vi "FPGAmain_v2.vi"() -> ()   [LabVIEW 2013]
uses:
  FPGA/DataMode.ctl
  FPGA/AcquireState.ctl
  FPGA/Input_5782/5782_states.ctl
  <vilib>/Platform/TimedLoop/XDataNode/timing_clust.ctl
  <vilib>/Platform/TimedLoop/XDataNode/nitl_modes.ctl
  <vilib>/Platform/TimedLoop/XDataNode/wakeup.ctl
  <vilib>/rvi/Emulation/niFpgaSctlEmulationGetInTimedLoop.vi
  <vilib>/rvi/Emulation/niFpgaEmulationReportErrorSimple.vi
  <vilib>/rvi/Emulation/niFpgaGetClockAttributes.vi
  <vilib>/rvi/eio/common/nirviEmuTemplateMethod_errors.vi
  <vilib>/rvi/Emulation/niFpgaCriticalErrorInLSC.vi
  <vilib>/rvi/FIFO/Fifo_Resource/nirvififoEmulationWriteFpgaImpl.vi
  <vilib>/rvi/DataTransferAndStorage/Container/Common/niFpgaContainerGetUniqueNameForEmu.vi
  <vilib>/rvi/FIFO/Fifo_Resource/nirvififoEmulationReadFpgaImpl.vi
  <vilib>/rvi/DataTransferAndStorage/Register/Emulation/niFpgaRegisterEmulationFpgaImpl.vi
  <instcachedir>/0/niFpgaRegisterEmulationFpgaImpl_DCF4BC0110594B98B44A971D60CEEC4D.lvgen/niFpgaRegisterEmulationFpgaImpl_DCF4BC0110594B98B44A971D60CEEC4D_016.vi
  <instcachedir>/0/niFpgaRegisterEmulationFpgaImpl_DCF4BC0110594B98B44A971D60CEEC4D.lvgen/niFpgaRegisterEmulationFpgaImpl_DCF4BC0110594B98B44A971D60CEEC4D_003.vi
  <instcachedir>/0/niFpgaRegisterEmulationFpgaImpl_DCF4BC0110594B98B44A971D60CEEC4D.lvgen/niFpgaRegisterEmulationFpgaImpl_DCF4BC0110594B98B44A971D60CEEC4D_014.vi
  <instcachedir>/0/niFpgaRegisterEmulationFpgaImpl_DCF4BC0110594B98B44A971D60CEEC4D.lvgen/niFpgaRegisterEmulationFpgaImpl_DCF4BC0110594B98B44A971D60CEEC4D_015.vi
  <vilib>/rvi/interface/RandomDataEmulation/nirviRandomDataMultiElementFPGAFIFO.vi
  <instcachedir>/0/nirviRandomDataMultiElementFPGAFIFO_F2B80EDE0D7944A08478D8D26097D4DB.lvgen/nirviRandomDataMultiElementFPGAFIFO_F2B80EDE0D7944A08478D8D26097D4DB_005.vi
  <vilib>/rvi/interface/RandomDataEmulation/niFpgaRandomDataHandleErrors.vi
  <vilib>/rvi/interface/RandomDataEmulation/nirviRandomDataFPGAFIFO.vi
  <instcachedir>/0/niFpgaRegisterEmulationFpgaImpl_DCF4BC0110594B98B44A971D60CEEC4D.lvgen/niFpgaRegisterEmulationFpgaImpl_DCF4BC0110594B98B44A971D60CEEC4D_009.vi
  <instcachedir>/0/niFpgaRegisterEmulationFpgaImpl_DCF4BC0110594B98B44A971D60CEEC4D.lvgen/niFpgaRegisterEmulationFpgaImpl_DCF4BC0110594B98B44A971D60CEEC4D_013.vi
  <vilib>/Platform/TimedLoop/XDataNode/XDataNode.xnode
  <vilib>/eio/EIONode/EIONode.xnode
  <vilib>/rvi/DataTransferAndStorage/Container/XNode/niFpgaContainer.xnode
  <vilib>/rvi/FIFO/Fifo_Resource/nirvififoEmulationWrite.vi
  <vilib>/rvi/FIFO/Fifo_Resource/nirvififoEmulationRead.vi
  <vilib>/rvi/DataTransferAndStorage/Register/Emulation/niFpgaRegisterEmulation.vi
  <vilib>/rvi/interface/RandomDataEmulation/nirviRandomDataFpgaMultiElementTemplate.vi
  <vilib>/rvi/interface/RandomDataEmulation/nirviRandomDataFpgaReadWriteTemplate.vi
  <vilib>/rvi/FIFO/Fifo_Resource/nirvififoEmulationP2P.vi
  <vilib>/Platform/TimedLoop/XDataNode/XDNodeRunTimeDep.lvlib
  <instrlib>/FlexRIO/Libraries/Helper VIs/NI FlexRIO Helper VIs.lvlib
panel:
  in  "delay phase":fxp<+,64,64>
  in  "AM phase":fxp<+,64,64>
  in  "Phase 5782":fxp<+,64,64>[](array[numeric])=[0.0, 0.0]
  in  "User Command Commit":bool
  in  "User Command":u8
  out "User Command Idle":bool
  out "User Command Status":u8
  in  "User Data 0":u8
  in  "User Data 1":u8
  out "PLL Locked":bool
  out "User Error":bool
  out "Configured?":bool
  in  "FIR coeffs":fxp<+/-,18,18>[](array[numeric])
  in  "Phase output":fxp<+,64,64>[](array[numeric])=[0.0, 0.0, 0.0, 0.0]
  in  "5782 record length":u16=4000 caption="Samples Per Trigger" min=1 step=1
  in  "Trigger Acquisition":bool
  in  "Continuous":bool
  out "IO Module\\Trigger Input":bool
  in  "Mode":T1
  in  "Simulated phase 5782":fxp<+,64,64>[](array[numeric])=[0.0, 0.0]
  in  "Acquisition running":bool
  in  "Samples Per Trigger":i32 min=1 step=1
  in  "Trigger simulated data":bool
  in  "simulated phase 5160":fxp<+,64,64>
  in  "phase 5160":fxp<+,64,64>
  # "Dynamic filter"
  # "Dynamic downsample"
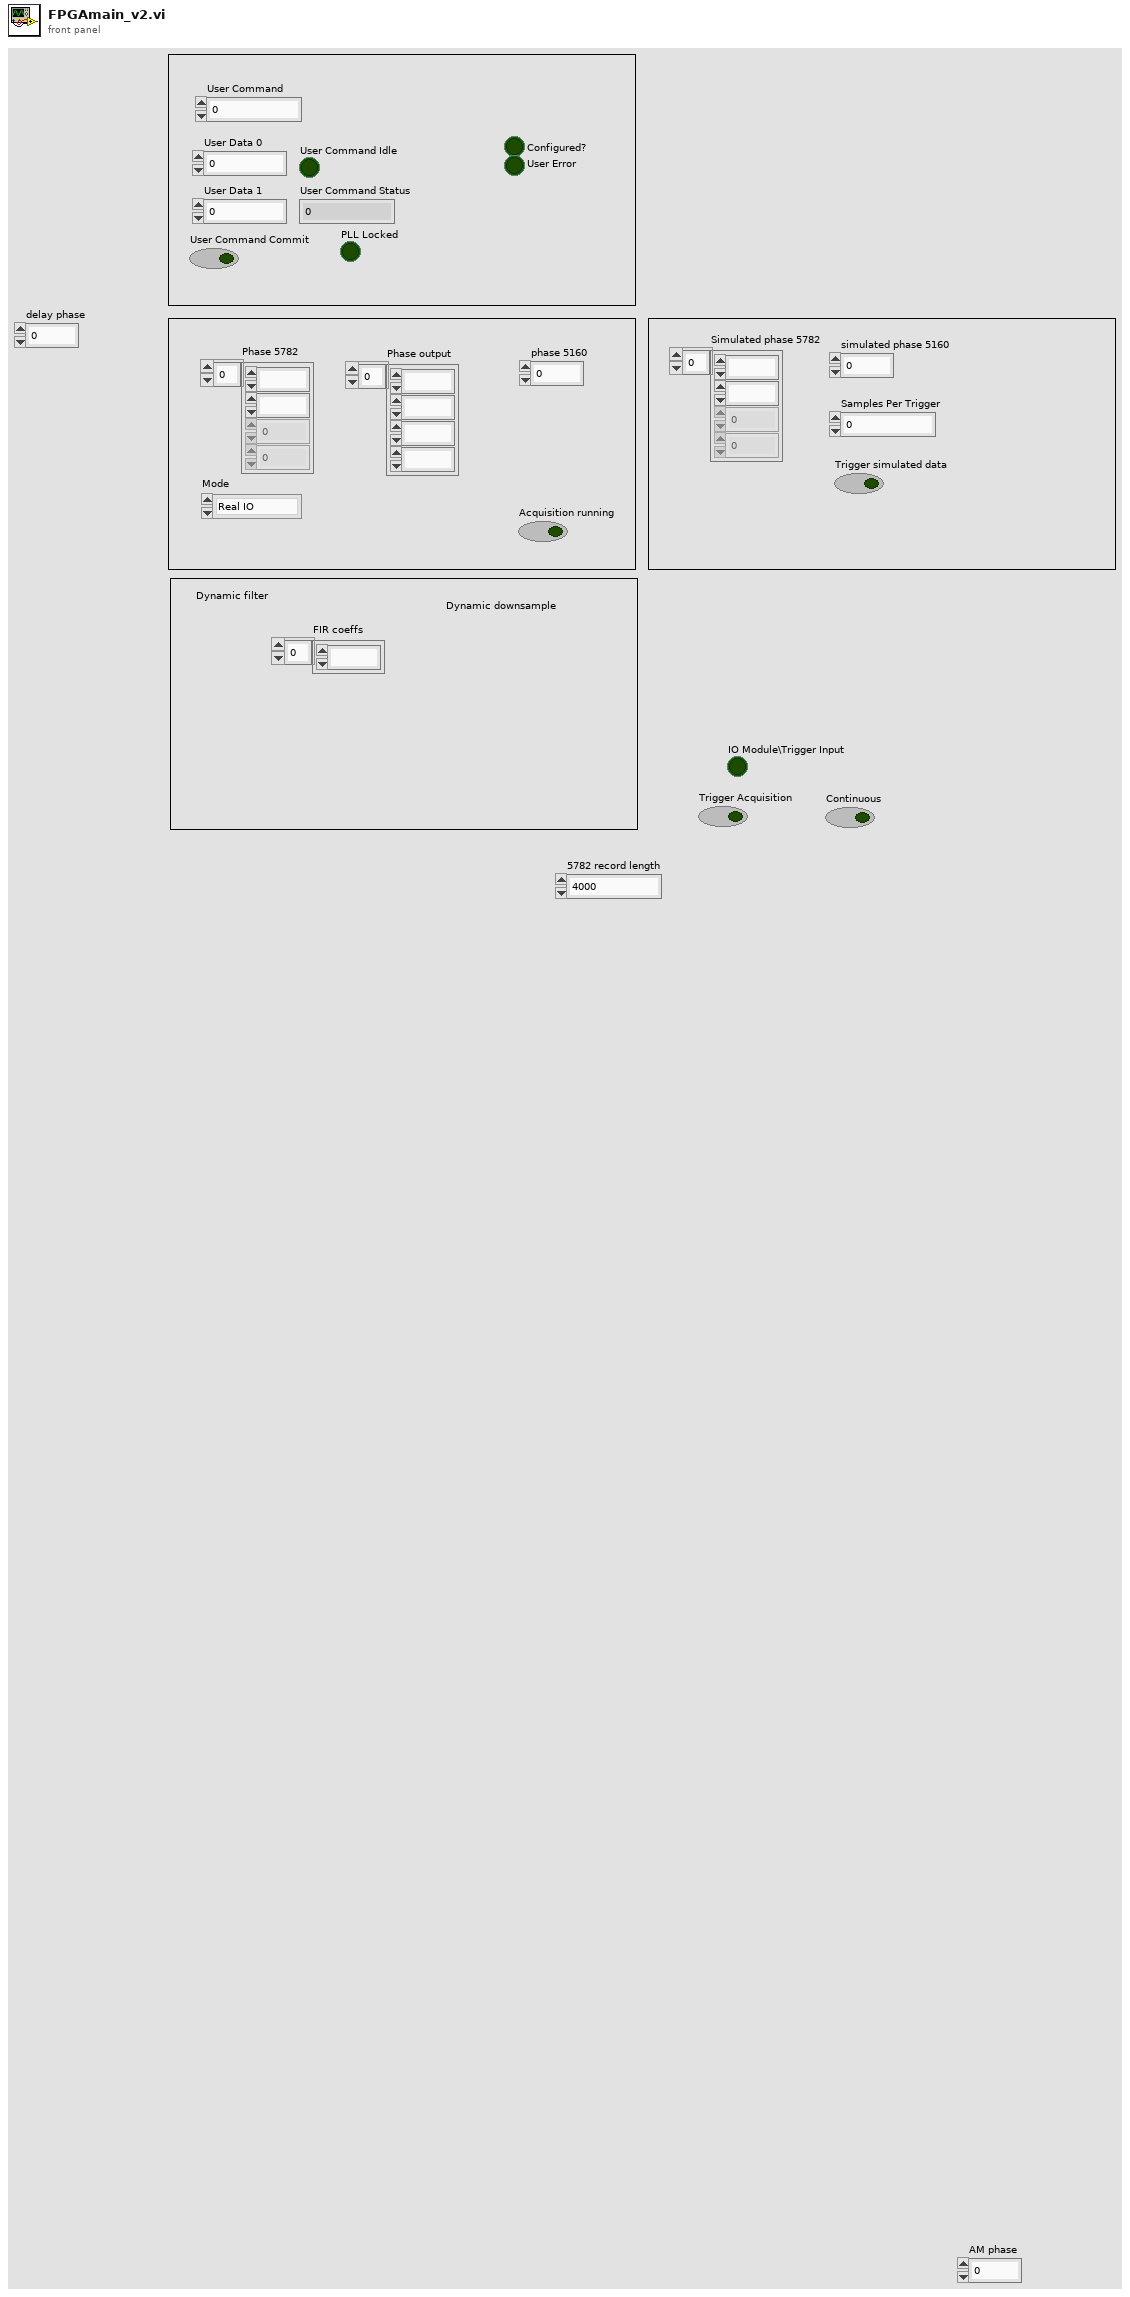
[diagram p1: front panel]
types:
  T1 = typedef "DataMode.ctl" = enum16{"Real IO", "Simulated"}
  T2 = typedef "5782_states.ctl" = enum8{"Wait for trigger", "Acquisition", "Send record length", "Quiet period"}
  T3 = typedef "AcquireState.ctl" = enum8{"Idle", "Acquire"}
  T4 = typedef "XDNodeRunTimeDep.lvlib/timing_clust.ctl" = cluster{"Expected End [f-1]":u64, "Actual End [f-1]":u64, "Finished Late? [f-1]":bool, "Expected End [i-1]":u64, "Actual End [i-1]":u64, "Finished Late? [i-1]":bool, "Expected Start [i]":u64, "Actual Start [i]":u64, "Expected Start [f]":u64, "Actual Start [f]":u64, "Source Name":string, "Structure Name":string, "Period":i64, "Deadline":i64, "Offset":i64, "Start":i64, "Priority":i32, "Timeout":i32, "Mode":T5, "Wakeup Reason":T6, "Error":errorcluster, "Source Type":string, "Secondary Source Type":string, "Global End Time":u64, "Global Start Time":u64, "Frame Duration":u64, "Iteration Duration":u64, "Assigned CPU":i32, "I/O Scan Engine Mode":u32}
  T5 = typedef "XDNodeRunTimeDep.lvlib/nitl_modes.ctl" = enum32{"No Change", "Process missed periods, maintain original phase", "Discard missed periods, maintain original phase", "Process missed periods, ignore original phase", "Discard missed periods, ignore original phase"}
  T6 = typedef "XDNodeRunTimeDep.lvlib/wakeup.ctl" = enum32{"Normal", "Aborted", "Asynchronous wakeup", "Timing source error", "Timed loop error", "Timeout"}
  T7 = typedef "I16 array size 2.ctl" = i16[]
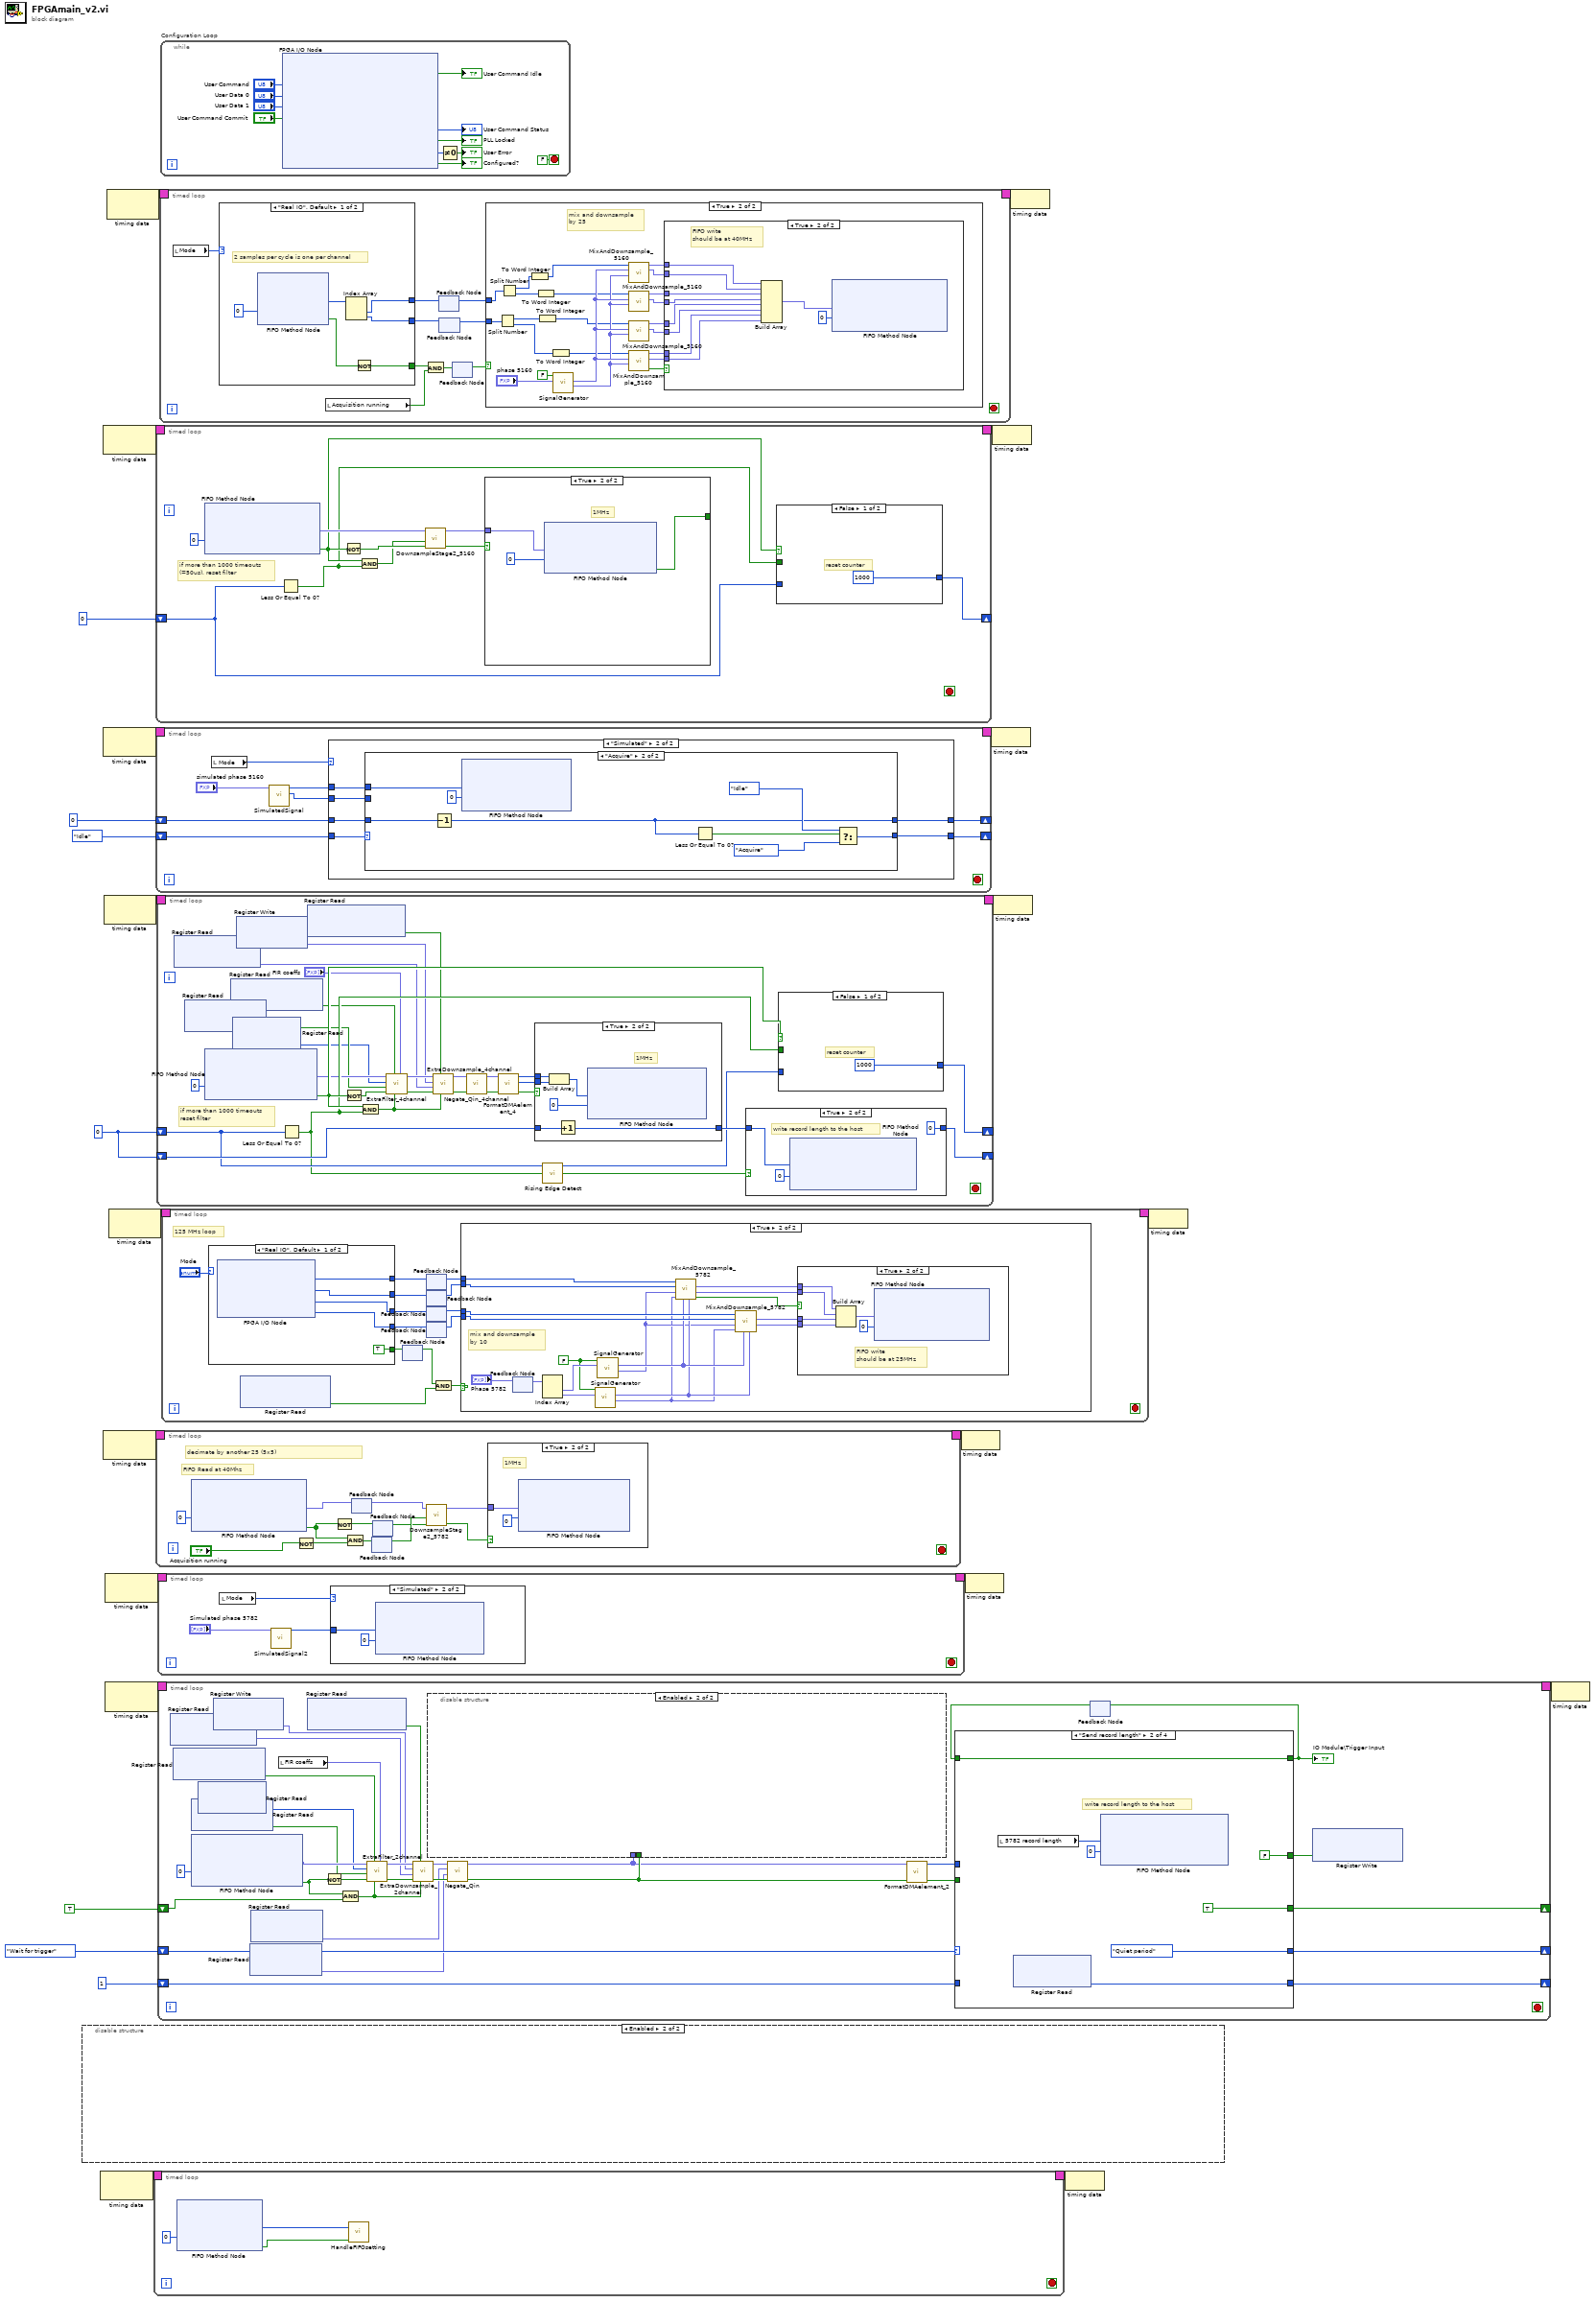
[diagram p0: block diagram]
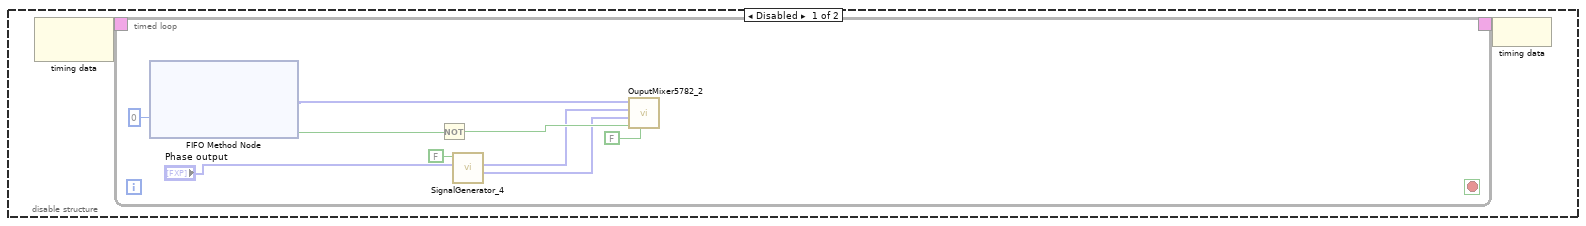
[diagram p2: hidden frame]
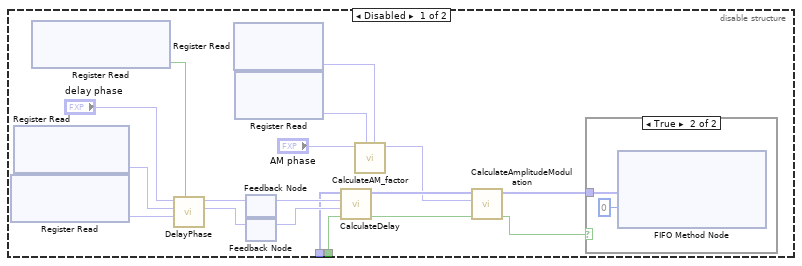
[diagram p3: hidden frame]
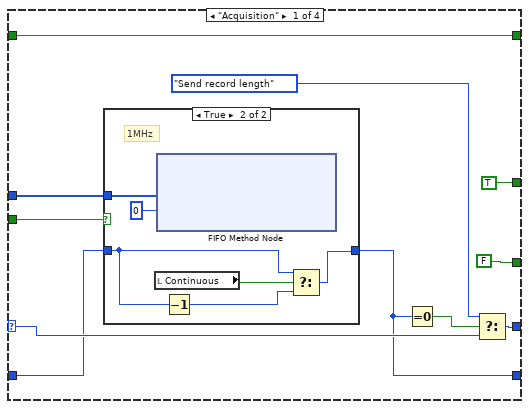
[diagram p5: hidden frame]
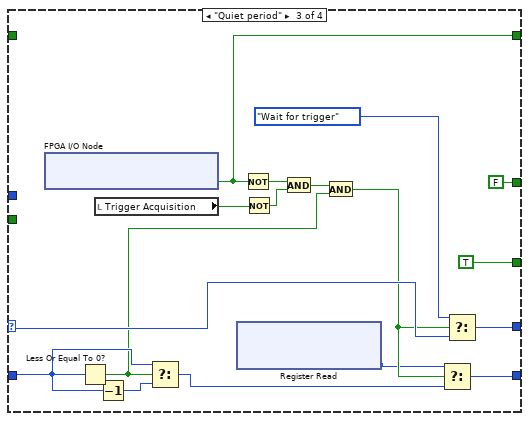
[diagram p7: hidden frame]
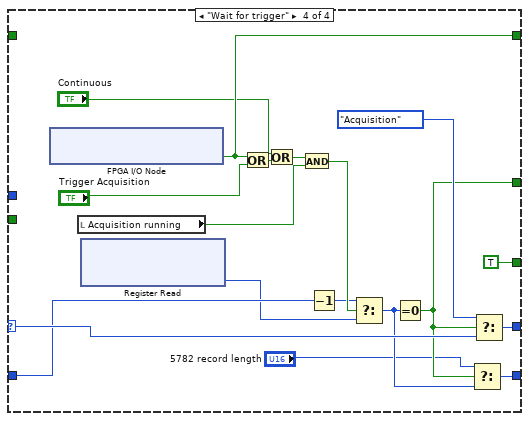
[diagram p8: hidden frame]
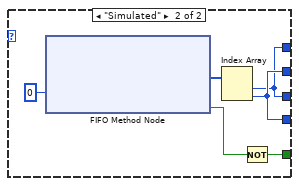
[diagram p11: hidden frame]
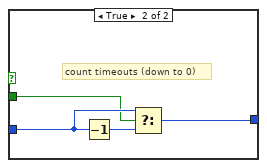
[diagram p14: hidden frame]
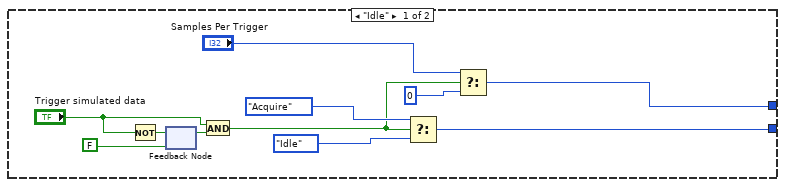
[diagram p18: hidden frame]
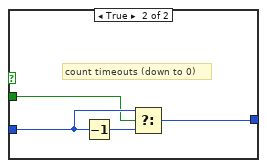
[diagram p19: hidden frame]
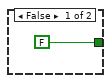
[diagram p20: hidden frame]
diagram:
  w14 = 0 ("y")
  n1 = disable-structure shown="Enabled" {
    frame Disabled {
      n2 = node-c288() -> (w27:T4)  [unwired: 1 in]
      n3 = timed-loop {
        timing: w27 -> [_]
        timing-out: [_] -> w26
        stop <- _ stop-if-true
        n4 = xnode ("FIFO Method Node")("Timeout"=0) -> ("Element"=w28:fxp<+/-,16,14>[], "Timed Out?"=w30:bool)  [unwired: 1 in, 1 out]
        n5 = Not(x=w30) -> (.not. x?=w34:bool)
        n6 = call "SignalGenerator_4.vi"("Phase"="Phase output", "reset"=FALSE) -> ("Sine out"=w31:fxp<+/-,16,0>[], "Cosine out"=w32:fxp<+/-,16,0>[])  [unwired: 8 in]
        n7 = call "OuputMixer5782_2.vi"("reset"=FALSE, "valid in"=w34, "Sine in"=w31, "Cosine in"=w32, "Data in"=w28) -> ()  [unwired: 5 in, 2 out]
      }
      n8 = node-c288(w26) -> ()
    }
    frame Enabled {
    }
  }
  n9 = node-c288() -> (w5:T4)  [unwired: 1 in]
  n10 = node-c288() -> (w23:T4)  [unwired: 1 in]
  n11 = node-c288() -> (w21:T4)  [unwired: 1 in]
  n12 = node-c288() -> (w11:T4)  [unwired: 1 in]
  n13 = node-c288() -> (w16:T4)  [unwired: 1 in]
  n14 = node-c288() -> (w13:T4)  [unwired: 1 in]
  n15 = node-c288() -> (w7:T4)  [unwired: 1 in]
  n16 = node-c288() -> (w25:T4)  [unwired: 1 in]
  n17 = node-c288() -> (w9:T4)  [unwired: 1 in]
  n18 = timed-loop {
    timing: w5 -> [_]
    timing-out: [_] -> w4
    stop <- _ stop-if-true
    n19 = xnode ("FIFO Method Node")("Timeout"=0) -> ("Element"=w42:u64, "Timed Out?"=w41:bool)  [unwired: 1 in, 1 out]
    n20 = call "HandleFIFOsetting.vi"("timed out"=w41, "Value"=w42) -> ()  [unwired: 10 in]
  }
  n21 = timed-loop {
    timing: w23 -> [_]
    timing-out: [_] -> w22
    shift-right: [w48] -> _
    shift-left: 0 ("y") -> [w47]
    stop <- _ stop-if-true
    # "if more than 1000 timeouts\n(=50us), reset filter"
    n22 = xnode ("FIFO Method Node")("Timeout"=0) -> ("Element"=w52:fxp<+/-,16,14>[], "Timed Out?"=w49:bool)  [unwired: 1 in, 1 out]
    n23 = Less Or Equal To 0?(x=w47) -> (x <= 0?=w46:bool)
    n24 = Not(x=w49) -> (.not. x?=w53:bool)
    n25 = And(x=w49, y=w46) -> (x .and. y?=w50:bool)
    n26 = call "DownsampleStage2_5160.vi"("valid in"=w53, "reset"=w50, "Element"=w52) -> ("valid out"=w54:bool, "Array"=w55:fxp<+/-,16,14>[])  [unwired: 7 in]
    n27 = case shown="True" w54 {
      tunnel: w55 -> [_ w62]
      tunnel: [FALSE ("Timed Out?") w63] -> _
      frame False {
      }
      frame True {
        # "1MHz"
        n28 = xnode ("FIFO Method Node")("Element"=w62, "Timeout"=0) -> ("Timed Out?"=w63:bool)  [unwired: 1 in, 1 out]
      }
    }
    n29 = case shown="False" w49 {
      tunnel: w46 -> [_ w58]
      tunnel: w47 -> [_ w59]
      tunnel: [1000 ("y") w57] -> w48
      frame False {
        # "reset counter"
      }
      frame True {
        # "count timeouts (down to 0)"
        n30 = Decrement(x=w59) -> (x-1=w60:i32)
        n31 = Select(t=w59, s=w58, f=w60) -> (s? t:f=w57:i32)
      }
    }
  }
  n32 = timed-loop {
    timing: w21 -> [_]
    timing-out: [_] -> w20
    shift-right: [w70] -> _
    shift-left: 0 ("f") -> [w69]
    shift-right: [w68] -> _
    shift-left: AcquireState."Idle" ("Acquire State") -> [w67]
    stop <- _ stop-if-true
    n33 = local read "Mode"() -> (w74:T1)
    n34 = call "SimulatedSignal.vi"("phase"="simulated phase 5160") -> ("cos output"=w72:i16, "Sample output"=w73:i16)  [unwired: 9 in]
    n35 = case shown="\"Simulated\"" w74 {
      tunnel: w73 -> [_ w82]
      tunnel: w72 -> [_ w77]
      tunnel: [w76 w81] -> w70
      tunnel: w69 -> [w76 w80]
      tunnel: [w75 w79] -> w68
      tunnel: w67 -> [w75 w78]
      frame "Real IO" {
      }
      frame "Simulated" {
        n36 = case shown="\"Acquire\"" w78 {
          tunnel: w80 -> [_ w98]
          tunnel: [w87 w97] -> w79
          tunnel: [w84 w96] -> w81
          tunnel: w82 -> [_ w95]
          tunnel: w77 -> [_ _]
          frame "Idle" {
            n37 = Not(x="Trigger simulated data") -> (.not. x?=w88:bool)
            n38 = feedback #1(FALSE) -> (w89:bool)
            n39 = feedback-in #1(w88) -> ()
            n40 = And(x="Trigger simulated data", y=w89) -> (x .and. y?=w83:bool)
            n41 = Select(t=AcquireState."Acquire" ("Acquire State"), s=w83, f=AcquireState."Idle" ("Acquire State")) -> (s? t:f=w87:T3)
            n42 = Select(t="Samples Per Trigger", s=w83, f=0) -> (s? t:f=w84:i32)
          }
          frame "Acquire" {
            n43 = Decrement(x=w98) -> (x-1=w96:i32)
            n44 = xnode ("FIFO Method Node")("Element"=w95, "Timeout"=0) -> ()  [unwired: 1 in, 2 out]
            n45 = Less Or Equal To 0?(x=w96) -> (x <= 0?=w100:bool)
            n46 = Select(t=AcquireState."Idle" ("Acquire State"), s=w100, f=AcquireState."Acquire" ("Acquire State")) -> (s? t:f=w97:T3)
          }
        }
      }
    }
  }
  n47 = timed-loop {
    timing: w11 -> [_]
    timing-out: [_] -> w10
    stop <- _ stop-if-true
    # "FIFO Read at 40Mhz"
    # "decimate by another 25 (5x5)"
    n48 = xnode ("FIFO Method Node")("Timeout"=0) -> ("Element"=w110:fxp<+/-,16,14>[], "Timed Out?"=w111:bool)  [unwired: 1 in, 1 out]
    n49 = Not(x="Acquisition running") -> (.not. x?=w112:bool)
    n50 = Not(x=w111) -> (.not. x?=w106:bool)
    n51 = And(x=w111, y=w112) -> (x .and. y?=w108:bool)
    n52 = feedback #2() -> (w109:fxp<+/-,16,14>[])  [unwired: 1 in]
    n53 = feedback-in #2(w110) -> ()
    n54 = feedback #3() -> (w107:bool)  [unwired: 1 in]
    n55 = feedback-in #3(w108) -> ()
    n56 = feedback #4() -> (w105:bool)  [unwired: 1 in]
    n57 = feedback-in #4(w106) -> ()
    n58 = call "DownsampleStage2_5782.vi"("valid in"=w105, "reset"=w107, "Data in"=w109) -> ("valid out"=w113:bool, "data out"=w114:fxp<+/-,16,14>[])  [unwired: 7 in]
    n59 = case shown="True" w113 {
      tunnel: w114 -> [_ w116]
      frame False {
      }
      frame True {
        # "1MHz"
        n60 = xnode ("FIFO Method Node")("Element"=w116, "Timeout"=0) -> ()  [unwired: 1 in, 2 out]
      }
    }
  }
  n61 = timed-loop {
    timing: w16 -> [_]
    timing-out: [_] -> w15
    shift-right: [w142] -> _
    shift-left: w14 -> [w141]
    shift-right: [w144] -> _
    shift-left: w14 -> [w146]
    stop <- _ stop-if-true
    # "if more than 1000 timeouts\nreset filter"
    n62 = xnode ("Register Read")() -> ("Data"=w123:fxp<+,8,8>)  [unwired: 1 in, 1 out]
    n63 = xnode ("Register Read")() -> ("Data"=w121:bool)  [unwired: 1 in, 1 out]
    n64 = xnode ("FIFO Method Node")("Timeout"=0) -> ("Element"=w137:fxp<+/-,16,14>[], "Timed Out?"=w143:bool)  [unwired: 1 in, 1 out]
    n65 = xnode ("Register Read")() -> ("Data"=w122:bool)  [unwired: 1 in, 1 out]
    n66 = xnode ("Register Read")() -> ("Data"=w120:i32)  [unwired: 1 in, 1 out]
    n67 = xnode ("Register Write")() -> ("Data"=w124:fxp<+/-,32,1>)  [unwired: 1 in, 1 out]
    n68 = Less Or Equal To 0?(x=w141) -> (x <= 0?=w140:bool)
    n69 = xnode ("Register Read")() -> ("Data"=w125:bool)  [unwired: 1 in, 1 out]
    n70 = Not(x=w143) -> (.not. x?=w136:bool)
    n71 = And(x=w143, y=w140) -> (x .and. y?=w138:bool)
    n72 = call "ExtraFilter_4channel.vi"(5:"new coeffs"="FIR coeffs", "reset"=w138, 7:"new coeffs"=w122, "valid in"=w136, "enable filter"=w121, "new shift"=w120, "Data in"=w137) -> ("valid out"=w127:bool, "Data out"=w128:fxp<+/-,16,14>[])  [unwired: 3 in]
    n73 = call "ExtraDownsample_4channel.vi"("reset"=w138, "Set downsample"=w125, "valid in"=w127, "Downsample"=w123, "CIC Gain"=w124, "Data in"=w128) -> ("valid out"=w129:bool, "Data out"=w132:fxp<+/-,16,14>[])  [unwired: 4 in]
    n74 = call "Negate_Qin_4channel.vi"("valid in"=w129, "Data in"=w132) -> ("valid out"=w130:bool, "Data out"=w131:fxp<+/-,16,14>[])  [unwired: 8 in]
    n75 = call "FormatDMAelement_4.vi"("valid in"=w130, "Data in"=w131) -> ("valid out"=w133:bool, "Element2"=w134:u64, "Element1"=w135:u64)  [unwired: 7 in]
    n76 = case shown="True" w133 {
      tunnel: w135 -> [_ w162]
      tunnel: w134 -> [_ w161]
      tunnel: w146 -> [w157 w159]
      tunnel: [w157 w158] -> w145
      frame False {
      }
      frame True {
        # "1MHz"
        n77 = Build Array(w162, w161) -> (w160:u64[])
        n78 = Increment(x=w159) -> (x+1=w158:i32)
        n79 = xnode ("FIFO Method Node")("Element"=w160, "Timeout"=0) -> ()  [unwired: 1 in, 2 out]
      }
    }
    n80 = call <instrlib>:"Rising Edge Detect.vi"("signal"=w140) -> ("edge detected"=w139:bool)  [unwired: 14 in]
    n81 = case shown="True" w139 {
      tunnel: w145 -> [w153 w154]
      tunnel: [w153 0 ("y")] -> w144
      frame False {
      }
      frame True {
        # "write record length to the host"
        n82 = xnode ("FIFO Method Node")("Element"=w154, "Timeout"=0) -> ()  [unwired: 1 in, 2 out]
      }
    }
    n83 = case shown="False" w143 {
      tunnel: w140 -> [_ w150]
      tunnel: w141 -> [_ w151]
      tunnel: [1000 ("y") w149] -> w142
      frame False {
        # "reset counter"
      }
      frame True {
        # "count timeouts (down to 0)"
        n84 = Decrement(x=w151) -> (x-1=w152:i32)
        n85 = Select(t=w151, s=w150, f=w152) -> (s? t:f=w149:i32)
      }
    }
  }
  n86 = timed-loop {
    timing: w13 -> [_]
    timing-out: [_] -> w12
    stop <- _ stop-if-true
    n87 = local read "Mode"() -> (w168:T1)
    n88 = call "SimulatedSignal2.vi"("Phase"="Simulated phase 5782") -> ("output"=w167:T7)  [unwired: 9 in, 1 out]
    n89 = case shown="\"Simulated\"" w168 {
      tunnel: w167 -> [_ w169]
      frame "Real IO", Default {
      }
      frame "Simulated" {
        n90 = xnode ("FIFO Method Node")("Element"=w169, "Timeout"=0) -> ()  [unwired: 1 in, 2 out]
      }
    }
  }
  n91 = timed-loop {
    timing: w7 -> [_]
    timing-out: [_] -> w6
    shift-right: [w201] -> _
    shift-left: 5782_states."Wait for trigger" ("5782 states") -> [w203]
    shift-right: [w200] -> _
    shift-left: u16 1 ("trigger samples") -> [w202]
    shift-right: [w189] -> _
    shift-left: TRUE -> [w192]
    stop <- _ stop-if-true
    n92 = xnode ("Register Read")() -> ("Data"=w179:fxp<+,8,8>)  [unwired: 1 in, 1 out]
    n93 = xnode ("Register Read")() -> ("Data"=w185:bool)  [unwired: 1 in, 1 out]
    n94 = xnode ("Register Read")() -> ("Data"=w180:bool)  [unwired: 1 in, 1 out]
    n95 = xnode ("FIFO Method Node")("Timeout"=0) -> ("Element"=w194:fxp<+/-,16,14>[], "Timed Out?"=w193:bool)  [unwired: 1 in, 1 out]
    n96 = xnode ("Register Read")() -> ("Data"=w181:i32)  [unwired: 1 in, 1 out]
    n97 = xnode ("Register Write")() -> ("Data"=w178:fxp<+/-,32,1>)  [unwired: 1 in, 1 out]
    n98 = xnode ("Register Read")() -> ("Data"=w183:fxp<+/-,16,14>)  [unwired: 1 in, 1 out]
    n99 = xnode ("Register Read")() -> ("Data"=w184:fxp<+/-,16,14>)  [unwired: 1 in, 1 out]
    n100 = local read "FIR coeffs"() -> (w177:fxp<+/-,18,18>[])
    n101 = xnode ("Register Read")() -> ("Data"=w182:bool)  [unwired: 1 in, 1 out]
    n102 = Not(x=w193) -> (.not. x?=w196:bool)
    n103 = And(x=w193, y=w192) -> (x .and. y?=w198:bool)
    n104 = call "ExtraFilter_2channel.vi"(5:"new coeffs"=w177, "reset"=w198, 7:"new coeffs"=w185, "valid in"=w196, "enable filter"=w180, "new shift"=w181, "Data in"=w194) -> ("valid out"=w197:bool, "Data out"=w195:fxp<+/-,16,14>[])  [unwired: 3 in]
    n105 = call "ExtraDownsample_2channel.vi"("reset"=w198, "Set downsample"=w182, "valid in"=w197, "Downsample"=w179, "CIC Gain"=w178, "Data in"=w195) -> ("valid out"=w186:bool, "Data out"=w187:fxp<+/-,16,14>[])  [unwired: 4 in]
    n106 = call "Negate_Qin.vi"("valid in"=w186, "DC offset chan 1"=w183, "DC offset chan 0"=w184, "Data in"=w187) -> ("valid out"=w174:bool, "Data out"=w173:fxp<+/-,16,14>[])  [unwired: 6 in]
    n107 = disable-structure shown="Enabled" {
      disable-tunnel: w173 -> [w214 _]
      disable-tunnel: w174 -> [w210 _]
      frame Disabled {
        n108 = xnode ("Register Read")() -> ("Data"=w205:fxp<+/-,16,0>)  [unwired: 1 in, 1 out]
        n109 = xnode ("Register Read")() -> ("Data"=w206:fxp<+/-,16,0>)  [unwired: 1 in, 1 out]
        n110 = xnode ("Register Read")() -> ("Data"=w207:bool)  [unwired: 1 in, 1 out]
        n111 = call "DelayPhase.vi"("Use fixed delay"=w207, "fixed cos_fi"=w205, "fixed sin fi"=w206, "delay phase"="delay phase") -> ("cos_fi"=w212:fxp<+/-,16,0>, "sin fi"=w213:fxp<+/-,16,0>)  [unwired: 6 in]
        n112 = xnode ("Register Read")() -> ("Data"=w209:fxp<+/-,16,2>)  [unwired: 1 in, 1 out]
        n113 = xnode ("Register Read")() -> ("Data"=w208:fxp<+/-,16,2>)  [unwired: 1 in, 1 out]
        n114 = feedback #5() -> (w221:fxp<+/-,16,0>)  [unwired: 1 in]
        n115 = feedback-in #5(w213) -> ()
        n116 = feedback #6() -> (w220:fxp<+/-,16,0>)  [unwired: 1 in]
        n117 = feedback-in #6(w212) -> ()
        n118 = call "CalculateDelay.vi"("input valid"=w210, "cos_fi"=w220, "sin fi"=w221, "Data in"=w214) -> ("output valid"=w218:bool, "Data out"=w219:fxp<+/-,16,14>[])  [unwired: 6 in]
        n119 = call "CalculateAM_factor.vi"("b_am"=w209, "a_am"=w208, "AM phase"="AM phase") -> ("AM_factor"=w215:fxp<+/-,16,2>)  [unwired: 7 in, 1 out]
        n120 = call "CalculateAmplitudeModulation.vi"("input valid"=w218, "AM_factor"=w215, "Data in"=w219) -> ("output valid"=w216:bool, "Data out"=w217:fxp<+/-,16,14>[])  [unwired: 7 in]
        n121 = case shown="True" w216 {
          tunnel: w217 -> [_ w222]
          frame False {
          }
          frame True {
            n122 = xnode ("FIFO Method Node")("Element"=w222, "Timeout"=0) -> ()  [unwired: 1 in, 2 out]
          }
        }
      }
      frame Enabled {
      }
    }
    n123 = call "FormatDMAelement_2.vi"("valid in"=w174, "Data in"=w173) -> ("valid out"=w190:bool, "Element"=w191:u64[])  [unwired: 8 in]
    n124 = feedback #7() -> (w176:bool)  [unwired: 1 in]
    n125 = case shown="\"Send record length\"" w203 {
      selector: w203 -> [w234 _ w264 w283]
      tunnel: w202 -> [w230 _ w252 w272]
      tunnel: [w233 5782_states."Quiet period" ("5782 states") w263 w282] -> w201
      tunnel: [w227 w242 w265 w281] -> w200
      tunnel: w191 -> [w228 _ _ _]
      tunnel: w190 -> [w229 _ _ _]
      tunnel: [FALSE TRUE TRUE TRUE] -> w189
      tunnel: [TRUE FALSE ("5782 triggered") FALSE ("5782 triggered") w276] -> w188
      tunnel: [w226 w243 w254 w275] -> w175
      tunnel: w176 -> [w226 w243 _ _]
      frame "Acquisition" {
        n126 = case shown="True" w229 {
          tunnel: w228 -> [_ w241]
          tunnel: [w235 w238] -> w227
          tunnel: w230 -> [w235 w236]
          frame False {
          }
          frame True {
            # "1MHz"
            n127 = local read "Continuous"() -> (w239:bool)
            n128 = xnode ("FIFO Method Node")("Element"=w241, "Timeout"=0) -> ()  [unwired: 1 in, 2 out]
            n129 = Decrement(x=w236) -> (x-1=w237:u16)
            n130 = Select(t=w236, s=w239, f=w237) -> (s? t:f=w238:u16)
          }
        }
        n131 = Equal To 0?(x=w227) -> (x = 0?=w231:bool)
        n132 = Select(t=5782_states."Send record length" ("5782 states"), s=w231, f=w234) -> (s? t:f=w233:T2)
      }
      frame "Send record length" {
        # "write record length to the host"
        n133 = local read "5782 record length"() -> (w245:u16)
        n134 = xnode ("Register Read")() -> ("Data"=w242:u16)  [unwired: 1 in, 1 out]
        n135 = xnode ("FIFO Method Node")("Element"=w245, "Timeout"=0) -> ()  [unwired: 1 in, 2 out]
      }
      frame "Quiet period" {
        n136 = xnode "FPGA I/O Node"() -> ("IO Module\\Trigger Input"=w254:bool)  [unwired: 1 in, 1 out]
        n137 = Less Or Equal To 0?(x=w252) -> (x <= 0?=w251:bool)
        n138 = local read "Trigger Acquisition"() -> (w260:bool)
        n139 = Decrement(x=w252) -> (x-1=w253:u16)
        n140 = Select(t=w252, s=w251, f=w253) -> (s? t:f=w250:u16)
        n141 = xnode ("Register Read")() -> ("Data"=w249:u16)  [unwired: 1 in, 1 out]
        n142 = Not(x=w254) -> (.not. x?=w259:bool)
        n143 = Not(x=w260) -> (.not. x?=w258:bool)
        n144 = And(x=w259, y=w258) -> (x .and. y?=w257:bool)
        n145 = And(x=w257, y=w251) -> (x .and. y?=w262:bool)
        n146 = Select(t=w249, s=w262, f=w250) -> (s? t:f=w265:u16)
        n147 = Select(t=5782_states."Wait for trigger" ("5782 states"), s=w262, f=w264) -> (s? t:f=w263:T2)
      }
      frame "Wait for trigger" {
        n148 = xnode "FPGA I/O Node"() -> ("IO Module\\Trigger Input"=w275:bool)  [unwired: 1 in, 1 out]
        n149 = local read "Acquisition running"() -> (w277:bool)
        n150 = xnode ("Register Read")() -> ("Data"=w269:u16)  [unwired: 1 in, 1 out]
        n151 = Or(x=w275, y="Trigger Acquisition") -> (x .or. y?=w271:bool)
        n152 = Or(x="Continuous", y=w271) -> (x .or. y?=w270:bool)
        n153 = And(x=w270, y=w277) -> (x .and. y?=w278:bool)
        n154 = Decrement(x=w272) -> (x-1=w273:u16)
        n155 = Select(t=w273, s=w278, f=w269) -> (s? t:f=w274:u16)
        n156 = Equal To 0?(x=w274) -> (x = 0?=w276:bool)
        n157 = Select(t="5782 record length", s=w276, f=w274) -> (s? t:f=w281:u16)
        n158 = Select(t=5782_states."Acquisition" ("5782 states"), s=w276, f=w283) -> (s? t:f=w282:T2)
      }
    }
    "IO Module\\Trigger Input" <- w175
    n159 = feedback-in #7(w175) -> ()
    n160 = xnode ("Register Write")("Data"=w188) -> ()  [unwired: 1 in, 1 out]
  }
  n161 = timed-loop {
    timing: w25 -> [_]
    timing-out: [_] -> w24
    stop <- _ stop-if-true
    n162 = local read "Mode"() -> (w289:T1)
    n163 = case shown="\"Real IO\", Default" w289 {
      tunnel: [w331 w337] -> w294
      tunnel: [w328 w334] -> w288
      tunnel: [w330 w337] -> w291
      frame "Real IO", Default {
        # "2 samples per cycle is one per channel"
        n164 = xnode ("FIFO Method Node")("Timeout"=0) -> ("Element"=w333:u32[], "Timed Out?"=w329:bool)  [unwired: 1 in, 1 out]
        n165 = Index Array(array=w333) -> (element #1=w331:u32, element #2=w330:u32)  [unwired: 2 in]
        n166 = Not(x=w329) -> (.not. x?=w328:bool)
      }
      frame "Simulated" {
        n167 = xnode ("FIFO Method Node")("Timeout"=0) -> ("Element"=w336:i16, "Timed Out?"=w335:bool)  [unwired: 1 in, 1 out]
        n168 = Not(x=w335) -> (.not. x?=w334:bool)
        n169 = Join Numbers(hi=w336, lo=w336) -> ((hi.lo)=w337:u32)
      }
    }
    n170 = local read "Acquisition running"() -> (w287:bool)
    n171 = And(x=w288, y=w287) -> (x .and. y?=w286:bool)
    n172 = feedback-in #8(w294) -> ()
    n173 = feedback #8() -> (w293:u32)  [unwired: 1 in]
    n174 = feedback #9() -> (w290:u32)  [unwired: 1 in]
    n175 = feedback-in #9(w291) -> ()
    n176 = feedback #10() -> (w292:bool)  [unwired: 1 in]
    n177 = feedback-in #10(w286) -> ()
    n178 = case shown="True" w292 {
      tunnel: w293 -> [_ w308]
      tunnel: w290 -> [_ w297]
      frame False {
        # "FIFO read timeout, no data"
      }
      frame True {
        # "mix and downsample\nby 25"
        n179 = Split Number(x=w297) -> (hi(x)=w298:u16, lo(x)=w299:u16)
        n180 = Split Number(x=w308) -> (hi(x)=w307:u16, lo(x)=w306:u16)
        n181 = To Word Integer(number=w307) -> (16bit integer=w301:i16)
        n182 = To Word Integer(number=w306) -> (16bit integer=w300:i16)
        n183 = To Word Integer(number=w298) -> (16bit integer=w295:i16)
        n184 = To Word Integer(number=w299) -> (16bit integer=w296:i16)
        n185 = call "SignalGenerator.vi"("phase"="phase 5160", "Reset"=FALSE) -> ("Cos"=w302:fxp<+/-,16,0>, "Sin"=w303:fxp<+/-,16,0>)  [unwired: 7 in, 1 out]
        n186 = call "MixAndDownsample_5160.vi"("Sine in"=w302, "Cosine in"=w303, "Sample in"=w301) -> ("Q out"=w315:fxp<+/-,16,14>, "I out"=w317:fxp<+/-,16,14>)  [unwired: 6 in, 1 out]
        n187 = call "MixAndDownsample_5160.vi"("Sine in"=w302, "Cosine in"=w303, "Sample in"=w300) -> ("Q out"=w313:fxp<+/-,16,14>, "I out"=w314:fxp<+/-,16,14>)  [unwired: 6 in, 1 out]
        n188 = call "MixAndDownsample_5160.vi"("Sine in"=w302, "Cosine in"=w303, "Sample in"=w295) -> ("Q out"=w311:fxp<+/-,16,14>, "I out"=w312:fxp<+/-,16,14>)  [unwired: 6 in, 1 out]
        n189 = call "MixAndDownsample_5160.vi"("Sine in"=w302, "Cosine in"=w303, "Sample in"=w296) -> ("valid out"=w316:bool, "Q out"=w309:fxp<+/-,16,14>, "I out"=w310:fxp<+/-,16,14>)  [unwired: 6 in]
        n190 = case shown="True" w316 {
          tunnel: w317 -> [_ w326]
          tunnel: w315 -> [_ w325]
          tunnel: w314 -> [_ w324]
          tunnel: w313 -> [_ w318]
          tunnel: w312 -> [_ w323]
          tunnel: w311 -> [_ w322]
          tunnel: w310 -> [_ w321]
          tunnel: w309 -> [_ w320]
          frame False {
          }
          frame True {
            # "FIFO write\nshould be at 40MHz"
            n191 = Build Array(w326, w325, w324, w318, w323, w322, w321, w320) -> (w319:fxp<+/-,16,14>[])
            n192 = xnode ("FIFO Method Node")("Element"=w319, "Timeout"=0) -> ()  [unwired: 1 in, 2 out]
          }
        }
      }
    }
  }
  n193 = while "Configuration Loop" {
    stop <- FALSE stop-if-true
    n194 = xnode "FPGA I/O Node"("IO Module\\User Command"="User Command", "IO Module\\User Data 0"="User Data 0", "IO Module\\User Data 1"="User Data 1", "IO Module\\User Command Commit"="User Command Commit") -> ("IO Module\\User Command Idle"=→"User Command Idle":bool, "IO Module\\User Command Status"=→"User Command Status":u8, "IO Module\\PLL Locked"=→"PLL Locked":bool, "IO Module\\User Error"=w346:u8, "IO Module\\Initialization Done"=→"Configured?":bool)  [unwired: 9 in, 9 out]
    n195 = Not Equal To 0?(x=w346) -> (x != 0?=→"User Error":bool)
  }
  n196 = timed-loop {
    timing: w9 -> [_]
    timing-out: [_] -> w8
    stop <- _ stop-if-true
    # "125 MHz loop"
    n197 = case shown="\"Real IO\", Default" "Mode" {
      tunnel: [w393 w396] -> w363
      tunnel: [w392 w397] -> w361
      tunnel: [w391 w396] -> w359
      tunnel: [w390 w397] -> w356
      tunnel: [TRUE w394] -> w355
      frame "Real IO", Default {
        n198 = xnode "FPGA I/O Node"() -> ("IO Module\\AI 0 N-1"=w393:i16, "IO Module\\AI 0 N"=w392:i16, "IO Module\\AI 1 N-1"=w391:i16, "IO Module\\AI 1 N"=w390:i16)  [unwired: 4 in, 4 out]
      }
      frame "Simulated" {
        n199 = xnode ("FIFO Method Node")("Timeout"=0) -> ("Element"=w398:i16[], "Timed Out?"=w395:bool)  [unwired: 1 in, 1 out]
        n200 = Index Array(array=w398) -> (element #1=w396:i16, element #2=w397:i16)  [unwired: 2 in]
        n201 = Not(x=w395) -> (.not. x?=w394:bool)
      }
    }
    n202 = xnode ("Register Read")() -> ("Data"=w353:bool)  [unwired: 1 in, 1 out]
    n203 = feedback #11() -> (w354:bool)  [unwired: 1 in]
    n204 = feedback-in #11(w355) -> ()
    n205 = feedback #12() -> (w362:i16)  [unwired: 1 in]
    n206 = feedback-in #12(w363) -> ()
    n207 = feedback #13() -> (w360:i16)  [unwired: 1 in]
    n208 = feedback-in #13(w361) -> ()
    n209 = feedback #14() -> (w358:i16)  [unwired: 1 in]
    n210 = feedback-in #14(w359) -> ()
    n211 = feedback #15() -> (w357:i16)  [unwired: 1 in]
    n212 = feedback-in #15(w356) -> ()
    n213 = And(x=w354, y=w353) -> (x .and. y?=w364:bool)
    n214 = case shown="True" w364 {
      tunnel: w362 -> [_ w377]
      tunnel: w360 -> [_ w376]
      tunnel: w358 -> [_ w375]
      tunnel: w357 -> [_ w374]
      frame False {
      }
      frame True {
        w370 = FALSE
        # "mix and downsample\nby 10"
        n215 = feedback #16() -> (w372:fxp<+,64,64>[])  [unwired: 1 in]
        n216 = feedback-in #16("Phase 5782") -> ()
        n217 = Index Array(array=w372) -> (element #1=w371:fxp<+,64,64>, element #2=w373:fxp<+,64,64>)  [unwired: 2 in]
        n218 = call "SignalGenerator.vi"("phase"=w373, "Reset"=w370) -> ("Cos"=w365:fxp<+/-,16,0>, "Sin"=w367:fxp<+/-,16,0>)  [unwired: 7 in, 1 out]
        n219 = call "SignalGenerator.vi"("phase"=w371, "Reset"=w370) -> ("Cos"=w366:fxp<+/-,16,0>, "Sin"=w368:fxp<+/-,16,0>)  [unwired: 7 in, 1 out]
        n220 = call "MixAndDownsample_5782.vi"("sin1"=w367, "sin0"=w368, "cos1"=w365, "cos0"=w366, "signal 1"=w376, "signal 0"=w377) -> ("data valid"=w380:bool, "Q out"=w381:fxp<+/-,16,14>, "I out"=w382:fxp<+/-,16,14>)  [unwired: 3 in]
        n221 = call "MixAndDownsample_5782.vi"("sin1"=w367, "sin0"=w368, "cos1"=w365, "cos0"=w366, "signal 1"=w374, "signal 0"=w375) -> ("Q out"=w378:fxp<+/-,16,14>, "I out"=w379:fxp<+/-,16,14>)  [unwired: 3 in, 1 out]
        n222 = case shown="True" w380 {
          tunnel: w381 -> [_ w388]
          tunnel: w382 -> [_ w385]
          tunnel: w379 -> [_ w384]
          tunnel: w378 -> [_ w383]
          frame False {
          }
          frame True {
            # "FIFO write\nshould be at 25MHz"
            n223 = Build Array(w385, w388, w384, w383) -> (w387:fxp<+/-,16,14>[])
            n224 = xnode ("FIFO Method Node")("Element"=w387, "Timeout"=0) -> ()  [unwired: 1 in, 2 out]
          }
        }
      }
    }
  }
  n225 = node-c288(w10) -> ()
  n226 = node-c288(w12) -> ()
  n227 = node-c288(w20) -> ()
  n228 = node-c288(w22) -> ()
  n229 = node-c288(w15) -> ()
  n230 = node-c288(w24) -> ()
  n231 = node-c288(w4) -> ()
  n232 = node-c288(w8) -> ()
  n233 = node-c288(w6) -> ()
